vi "Get Info.vi"(8 "error in (no error)":errorcluster, 11 "IInfoable in":refnum<class "IInfoable.lvclass">) -> (0 "error out":errorcluster, 2 "Account Information":T1, 3 "IInfoable out":refnum<class "IInfoable.lvclass">)   [LabVIEW 2020, in "IInfoable.lvclass"]
uses:
  IInfoable.lvclass
  Account Information STYP.ctl
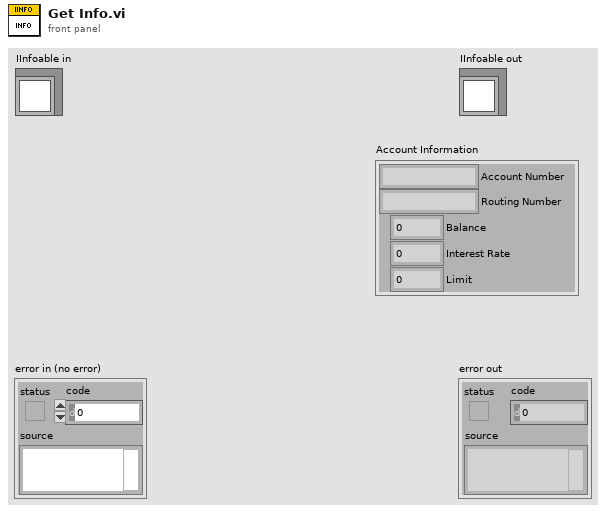
[diagram p1: front panel]
types:
  T1 = typedef "IInfoable.lvclass/Account Information STYP.ctl" = cluster{"Account Number":string, "Routing Number":string, "Balance":dbl, "Interest Rate":dbl, "Limit":dbl}
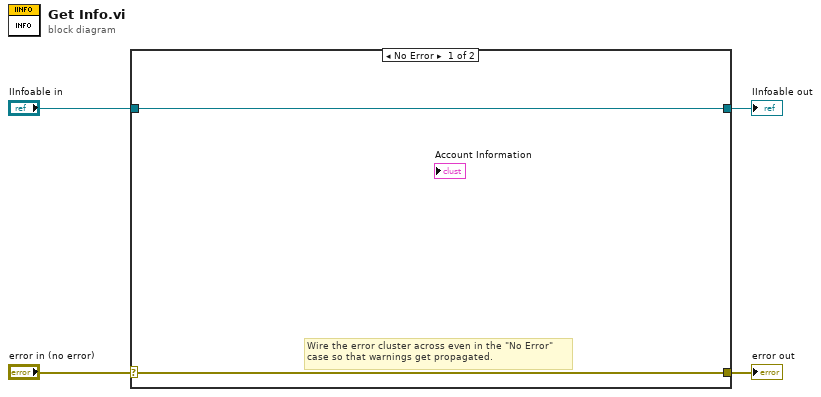
[diagram p0: block diagram]
diagram:
  n1 = case shown="No Error" "error in (no error)" {
    selector: "error in (no error)" -> [w5 w8]
    tunnel: [w5 w8] -> w3
    tunnel: [w6 w7] -> w1
    tunnel: "IInfoable in" -> [w6 w7]
    frame No Error {
      # "Wire the error cluster across even in the \"No Error\"\ncase so that warnings get propagated."
    }
    frame Error {
    }
  }
  "error out" <- w3
  "IInfoable out" <- w1
